vi "PMpara2Cpara.vi"(0 "PM para":T1(array[cluster]), 1 "Resolution multiple":dbl) -> (2 "cell para":sgl[][](array[numeric]))   [LabVIEW 2016]
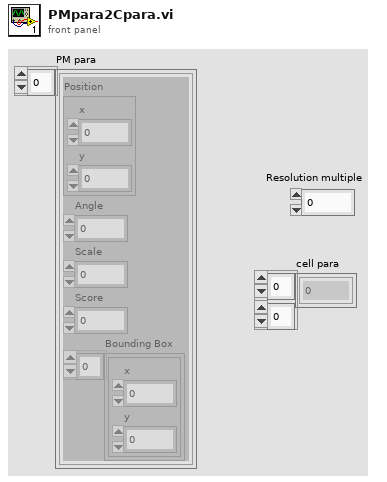
[diagram p1: front panel]
types:
  T1 = cluster{"Position":cluster{"x":sgl, "y":sgl}, "Angle":sgl, "Scale":sgl, "Score":sgl, "Bounding Box":cluster{"x":sgl, "y":sgl}[]}[]
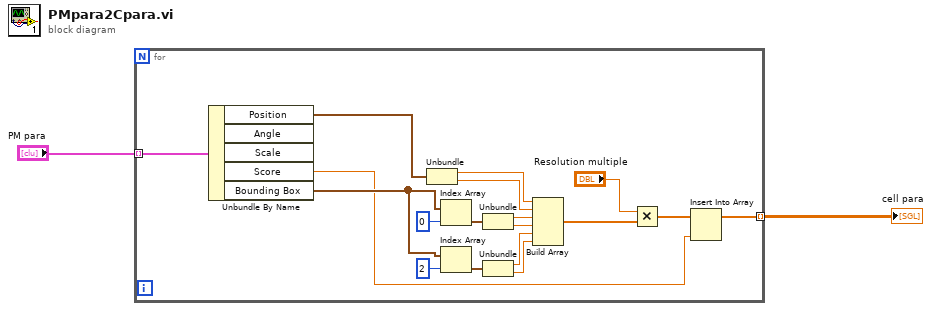
[diagram p0: block diagram]
diagram:
  n1 = for {
    tunnel: [w4] -> w1 mode=indexing
    tunnel: "PM para" -> [w8] mode=indexing
    n2 = Unbundle By Name(w8) -> ("Position"=w9:cluster{"x":sgl, "y":sgl}, "Score"=w6:sgl, "Bounding Box"=w20:cluster{"x":sgl, "y":sgl}[])  [unwired: 2 out]
    n3 = Unbundle(w9) -> ("x"=w14:sgl, "y"=w15:sgl)
    n4 = Index Array(array=w20, index=0 ("索引")) -> (element=w12:cluster{"x":sgl, "y":sgl})
    n5 = Index Array(array=w20, index=2 ("索引")) -> (element=w13:cluster{"x":sgl, "y":sgl})
    n6 = Unbundle(w12) -> ("x"=w16:sgl, "y"=w17:sgl)
    n7 = Unbundle(w13) -> ("x"=w18:sgl, "y"=w19:sgl)
    n8 = Build Array(w14, w15, w16, w17, w18, w19) -> (w7:sgl[])
    n9 = Multiply(x="Resolution multiple", y=w7) -> (x*y=w5:dbl[])
    n10 = Insert Into Array(array=w5, new element=w6) -> (w4:dbl[])  [unwired: 1 in]
  }
  "cell para" <- w1
